vi "Drive Auto Aim.vi"(8 "Auto Aim":bool, 10 "Right Axis 2":dbl, 11 "Left Axis 2":dbl) -> (2 "Right Axis":dbl, 3 "Left Axis":dbl)   [LabVIEW 2016]
uses:
  <vilib>/Rock Robotics/Network Tables/NT Read Number.vi
  Robot Global Data.vi
  <vilib>/Analysis/BLAS.llb/dnrm2 - Vector 2-Norm (DBL).vi
  <vilib>/addons/control/pid/pid.llb/PID Control Input Filter (DBL).vi
  <vilib>/Analysis/NI_AALBLAS.lvlib
  <vilib>/addons/control/pid/NI_PID_pid.lvlib
panel:
  in  "y deadzone":dbl
  out "distance x":dbl
  out "distance":dbl
  out "Delta Y middle goal":dbl
  in  "Final Align":cluster{"Kp":dbl, "Ki":dbl, "Kd":dbl}={"Kp"=0.01, "Ki"=0.0, "Kd"=0.0}
  in  "Deadzone":dbl format="%#_13g"
  in  "y":dbl=10.0 format="%#_13g"
  in  "v":dbl=0.7
  in  "Alpha":dbl=0.3
  out "Robot Position":cluster{dbl[], dbl[]}[](graph)
  out "roboRIO input voltage (V)":dbl
  out "angle diff":dbl
  in  "PID Gains":cluster{"Kp":dbl, "Ki":dbl, "Kd":dbl}={"Kp"=0.005, "Ki"=0.0, "Kd"=0.0}
  in  "reinitialize? (F)":bool
  in  "ff Angle comp":dbl=0.2
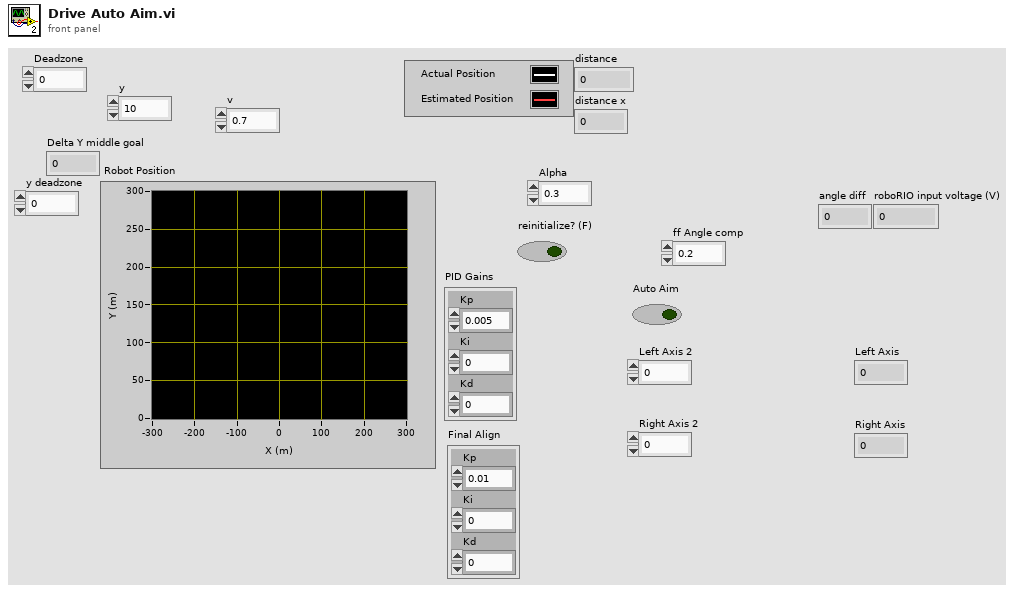
[diagram p1: front panel]
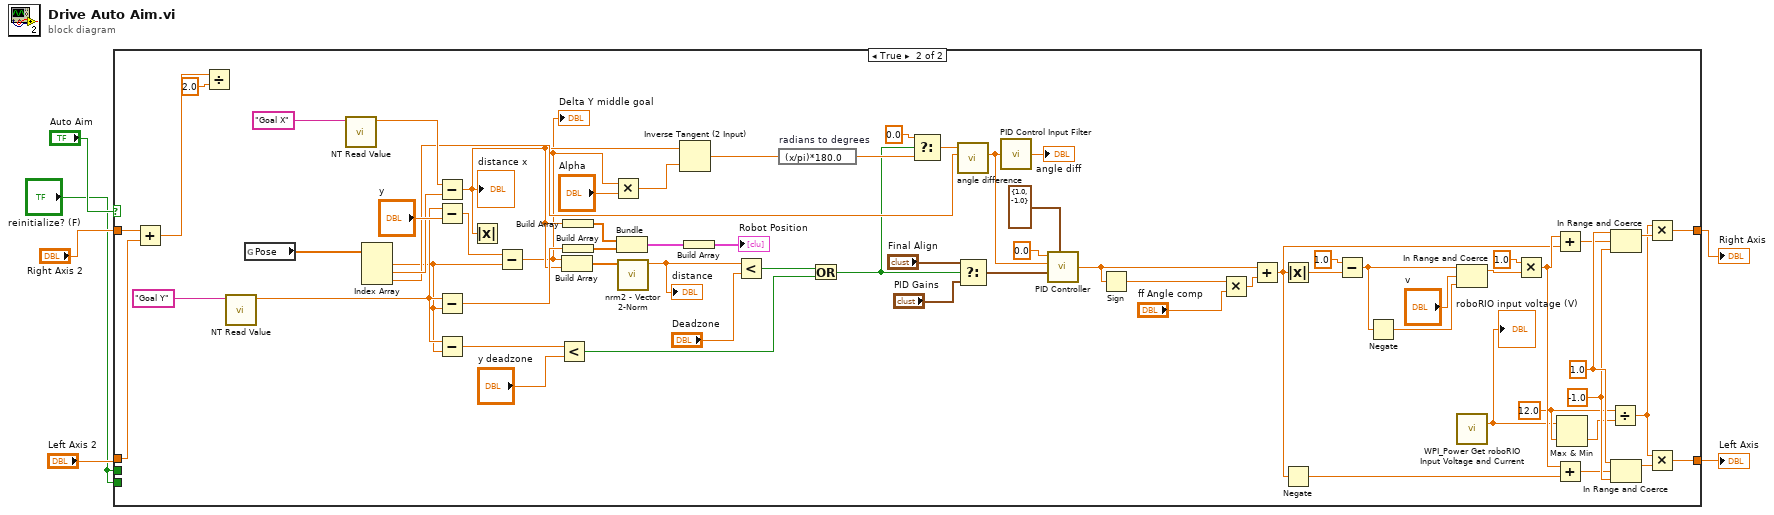
[diagram p0: block diagram]
diagram:
  n1 = case shown="True" "Auto Aim" {
    tunnel: [w7 w52] -> w2
    tunnel: [w8 w55] -> w1
    tunnel: "Right Axis 2" -> [w8 w35]
    tunnel: "Left Axis 2" -> [w7 w34]
    tunnel: "reinitialize? (F)" -> [_ _]
    tunnel: "reinitialize? (F)" -> [_ _]
    frame False {
    }
    frame True {
      w58 = 12.0 ("y")
      w75 = -1.0 ("upper limit")
      w76 = 1.0 ("upper limit")
      n2 = Add(x=w35, y=w34) -> (x+y=w33:dbl)
      n3 = Divide(x=w33, y=2.0) -> ()  [unwired: 1 out]
      n4 = call-poly <vilib>:"NT Read Value.vi"("Name"="Goal Y") -> ("Numeric"=w18:dbl)  [unwired: 9 in, 1 out]
      n5 = global read "Robot Global Data.vi" "Pose"() -> (w49:dbl[])
      n6 = call-poly <vilib>:"NT Read Value.vi"("Name"="Goal X") -> ("Numeric"=w46:dbl)  [unwired: 9 in, 1 out]
      n7 = Index Array(array=w49) -> (element #1=w17:dbl, element #2=w44:dbl, element #3=w43:dbl)  [unwired: 3 in]
      n8 = Subtract(x=w46, y=w44) -> (x-y=w11:dbl)
      "distance x" <- w11
      n9 = Subtract(x=w18, y="y") -> (x-y=w23:dbl)
      n10 = Subtract(x=w18, y=w17) -> (x-y=w21:dbl)
      n11 = Subtract(x=w18, y=w17) -> (x-y=w16:dbl)
      n12 = Absolute Value(x=w11) -> ()  [unwired: 1 out]
      n13 = Subtract(x=w23, y=w17) -> (x-y=w10:dbl)
      "Delta Y middle goal" <- w10
      n14 = Less?(x=w16, y="y deadzone") -> (x < y?=w14:bool)
      n15 = Build Array(w10, w11) -> (w45:dbl[])
      n16 = Build Array(w11) -> (w42:dbl[])
      n17 = Build Array(w21) -> (w41:dbl[])
      n18 = Multiply(x=w10, y="Alpha") -> (x*y=w9:dbl)
      n19 = Bundle(w42, w41) -> (w40:cluster{dbl[], dbl[]})  [unwired: 1 in]
      n20 = call-poly <vilib>:"nrm2 - Vector 2-Norm.vi"("x"=w45) -> ("dnrm2"=w20:dbl)  [unwired: 9 in, 1 out]
      "distance" <- w20
      n21 = Inverse Tangent (2 Input)(1:w9, 2:w11) -> (0:w13:dbl)
      n22 = Build Array(w40) -> (→"Robot Position":cluster{dbl[], dbl[]}[])
      n23 = Less?(x=w20, y="Deadzone") -> (x < y?=w19:bool)
      n24 = expression code="(x/pi)*180.0" "radians to degrees"(w13) -> (w27:dbl)
      n25 = Or(x=w19, y=w14) -> (x .or. y?=w12:bool)
      n26 = Select(t=0.0 ("f"), s=w12, f=w27) -> (s? t:f=w29:dbl)
      n27 = call "angle difference.vi"("angle2"=w43, "angle1"=w29) -> ("angle diff"=w37:dbl)  [unwired: 9 in]
      n28 = Select(t="Final Align", s=w12, f="PID Gains") -> (s? t:f=w24:cluster{"Kp":dbl, "Ki":dbl, "Kd":dbl})
      n29 = call-poly <vilib>:"PID Control Input Filter.vi"("input"=w37) -> ("output"=→"angle diff":dbl)  [unwired: 4 in]
      n30 = call "PID Controller.vi"("setpoint"=0.0, "process variable"=w37, "PID Gains"=w24, "Constrain"=cluster{"Max Control":dbl, "Min Control":dbl} {"Max Control"=1.0, "Min Control"=-1.0}) -> ("Control Signal"=w22:dbl)  [unwired: 1 in]
      n31 = Sign(1:w22) -> (0:w68:dbl)
      n32 = Multiply(x=w68, y="ff Angle comp") -> (x*y=w67:dbl)
      n33 = Add(x=w22, y=w67) -> (x+y=w66:dbl)
      n34 = Absolute Value(x=w66) -> (abs(x)=w64:dbl)
      n35 = Negate(x=w66) -> (-x=w73:dbl)
      n36 = Subtract(x=1.0, y=w64) -> (x-y=w63:dbl)
      n37 = Negate(x=w63) -> (-x=w62:dbl)
      n38 = In Range and Coerce(upper limit=w63, x="v", lower limit=w62) -> (coerced(x)=w71:dbl)  [unwired: 1 out]
      n39 = call <vilib>:"WPI_Power Get roboRIO Input Voltage and Current.vi"() -> ("roboRIO input voltage (V)"=w51:dbl)  [unwired: 13 in, 2 out]
      "roboRIO input voltage (V)" <- w51
      n40 = Multiply(x=1.0, y=w71) -> (x*y=w70:dbl)
      n41 = Add(x=w70, y=w66) -> (x+y=w74:dbl)
      n42 = Add(x=w70, y=w73) -> (x+y=w72:dbl)
      n43 = Max & Min(x=w51, y=w58) -> (min(x,y)=w57:dbl)  [unwired: 1 out]
      n44 = Divide(x=w58, y=w57) -> (x/y=w54:dbl)
      n45 = In Range and Coerce(upper limit=w76, x=w74, lower limit=w75) -> (coerced(x)=w56:dbl)  [unwired: 1 out]
      n46 = In Range and Coerce(upper limit=w76, x=w72, lower limit=w75) -> (coerced(x)=w53:dbl)  [unwired: 1 out]
      n47 = Multiply(x=w54, y=w56) -> (x*y=w55:dbl)
      n48 = Multiply(x=w54, y=w53) -> (x*y=w52:dbl)
    }
  }
  "Left Axis" <- w2
  "Right Axis" <- w1
